vi "get_distance.vi"(11 "NXT":T1={"Hardware"="NXT", "Flattened String"=""}) -> (0 "Distance (cm)":dbl, 3 "NXT 2":T1={"Hardware"="NXT", "Flattened String"=""})   [LabVIEW 2012]
uses:
  <vilib>/NXT/Subs/LVHSConnector.ctl
  <vilib>/NXT/Block Support/NXT_InputPort.ctl
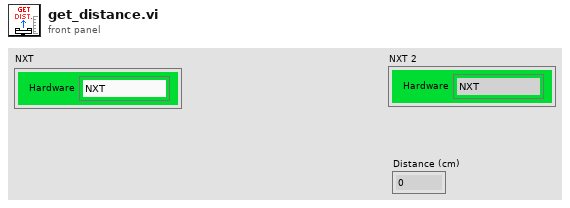
[diagram p1: front panel]
types:
  T1 = typedef "LVHSConnector.ctl" = cluster{"Hardware":string, "Flattened String":string}
  T2 = typedef "NXT_InputPort.ctl" = u8
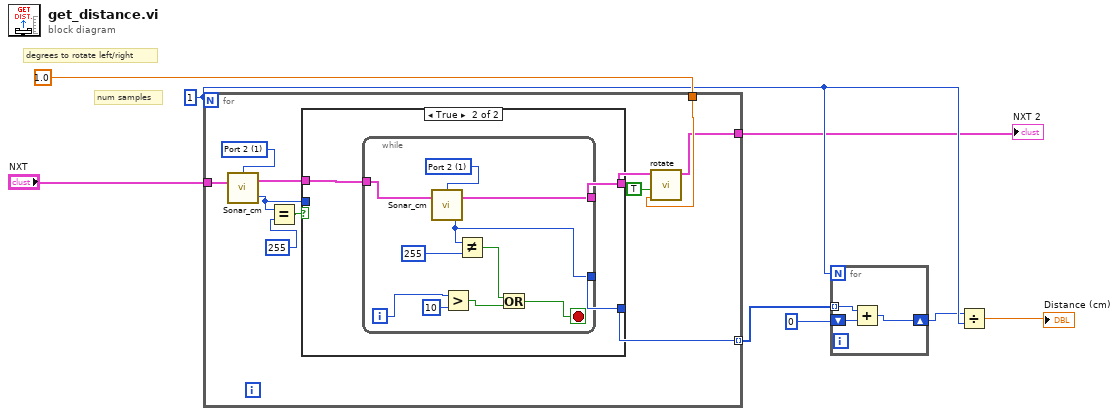
[diagram p0: block diagram]
diagram:
  w4 = 1 ("Angle of Rotation (360)")
  # "num samples"
  # "degrees to rotate left/right"
  n1 = for {
    N: w4 -> [_]
    tunnel: [w18] -> w6 mode=indexing
    tunnel: 1.0 ("degrees to  rotate") -> [w15]
    tunnel: [w14] -> w2
    tunnel: "NXT" -> [w13]
    w10 = T2 1 items=["Port 1", "Port 2", "Port 3", "Port 4"] ("Port (Port 4)")
    n2 = call <vilib>:"Sonar_cm.vi"("NXT"=w13, "Port (Port 4)"=w10) -> ("Distance (cm)"=w9:i16, "NXT"=w12:T1)  [unwired: 1 in]
    n3 = Equal?(x=w9, y=255 ("Angle of Rotation (360)")) -> (x = y?=w19:bool)
    n4 = case shown="True" w19 {
      tunnel: [w21 w24] -> w18
      tunnel: [w20 w22] -> w17
      tunnel: w12 -> [w20 w23]
      tunnel: w9 -> [w21 _]
      frame False {
      }
      frame True {
        n5 = while {
          tunnel: [w28] -> w24
          tunnel: w23 -> [w26]
          tunnel: [w25] -> w22
          i -> [w33]
          stop <- w31 stop-if-true
          w27 = T2 1 items=["Port 1", "Port 2", "Port 3", "Port 4"] ("Port (Port 4)")
          n6 = call <vilib>:"Sonar_cm.vi"("NXT"=w26, "Port (Port 4)"=w27) -> ("Distance (cm)"=w28:i16, "NXT"=w25:T1)  [unwired: 1 in]
          n7 = Greater?(x=w33, y=10 ("Angle of Rotation (360)")) -> (0:w32:bool)
          n8 = Not Equal?(x=w28, y=255 ("Angle of Rotation (360)")) -> (x != y?=w30:bool)
          n9 = Or(x=w30, y=w32) -> (x .or. y?=w31:bool)
        }
      }
    }
    n10 = call "rotate.vi"("degrees to  rotate"=w15, "right(T)/left(F)"=TRUE, "NXT 2"=w17) -> ("NXT"=w14:T1)  [unwired: 8 in]
  }
  "NXT 2" <- w2
  n11 = for {
    N: w4 -> [_]
    tunnel: w6 -> [w37] mode=indexing
    shift-right: [w35] -> w3
    shift-left: 0 ("Angle of Rotation (360)") -> [w36]
    n12 = Add(x=w37, y=w36) -> (x+y=w35:i32)
  }
  n13 = Divide(x=w3, y=w4) -> (x/y=→"Distance (cm)":dbl)
